vi "Write metadata to tiff string.vi"(8 "error in":errorcluster, 10 "Tiff image (unsigned byte array)":u8[](array[numeric]), 11 "Metadata string\n(must be at least 5 char long)":string) -> (0 "error out":errorcluster, 2 "Tiff file out (unsigned byte array)":u8[](array[numeric]))   [LabVIEW 2013, in "Tiff reader.lvlib"]
doc: "This .vi adds metadata to the tiff file (represented as a string)."
uses:
  Tiff reader.lvlib
  IFD Entry.ctl
  FieldTypes.ctl
  Long word to bytes.vi
panel:
  out "Time elapsed (ms)":u32
  out "Tag already exists?":bool
  out "Tag for metadata":T1
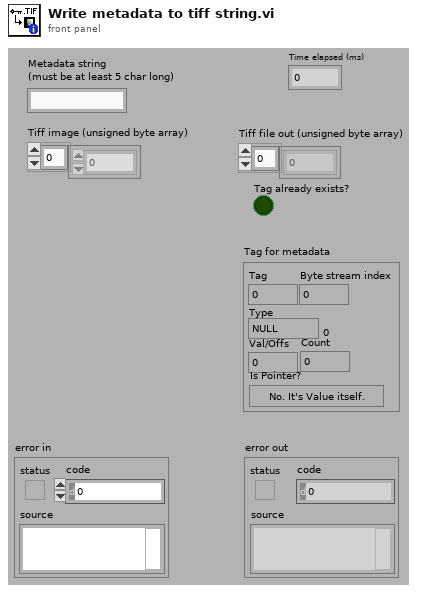
[diagram p1: front panel]
types:
  T1 = typedef "Tiff reader.lvlib/IFD Entry.ctl" = cluster{"Tag":u16, "Type":T2, "Count":u32, "Val/Offs":u32, "Is Pointer?":bool, "Byte stream index":i32}
  T2 = typedef "Tiff reader.lvlib/FieldTypes.ctl" = enum16{"NULL", "U8", "ASCII7", "U16", "U32", "RATIONAL", "SByte(I8)", "Undef(8Bit)", "I16", "I32", "SRat(4B:4B)", "SGL(4Byte)", "DBL(8Byte)"}
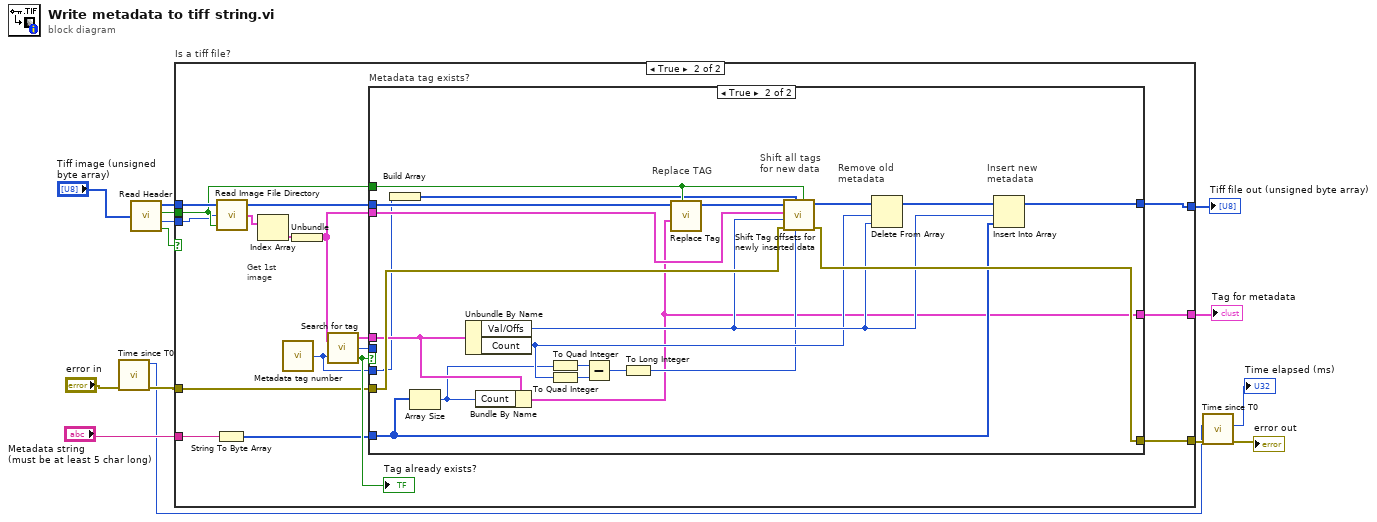
[diagram p0: block diagram]
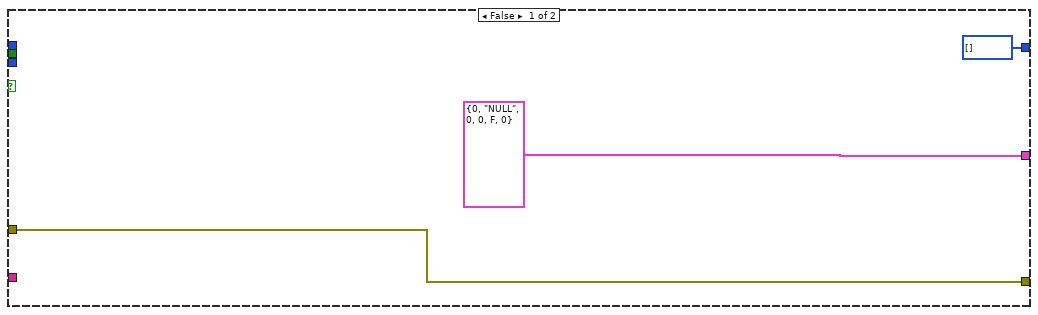
[diagram p2: hidden frame]
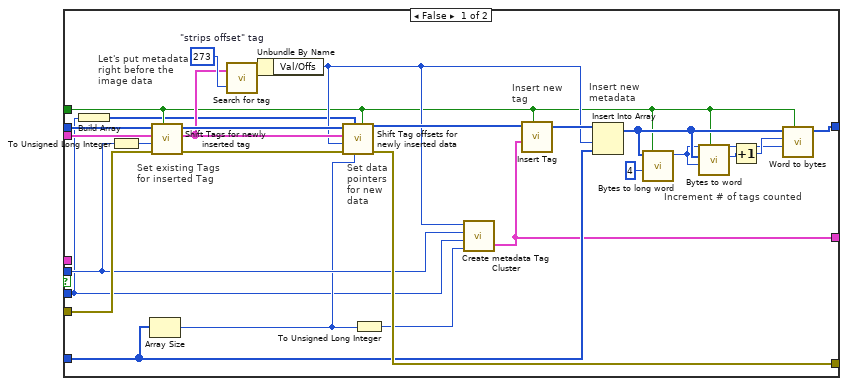
[diagram p3: hidden frame]
diagram:
  n1 = call "Time since T0.vi"("error in (no error)"="error in") -> ("error out"=w6:errorcluster, "current ms"=w2:u32)  [unwired: 2 in, 3 out]
  n2 = call "Read Header.vi"("TIFF Data in"="Tiff image (unsigned byte array)") -> ("TIFF Data out"=w13:u8[], "Litt/BigEnd"=w12:bool, "ImFileDirectOffs"=w14:u32, "IsTIFF?"=w11:bool)
  n3 = case "Is a tiff file?" shown="True" w11 {
    tunnel: w14 -> [_ w24]
    tunnel: w13 -> [_ w33]
    tunnel: [u8[] [] ("Image Data Out") w18] -> w9
    tunnel: w12 -> [_ w29]
    tunnel: "Metadata string\n(must be at least 5 char long)" -> [_ w27]
    tunnel: [T1 {"Tag"=0, "Type"=enum."NULL", "Count"=0, "Val/Offs"=0, "Is Pointer?"=FALSE, "Byte stream index"=0} ("Tag found") w25] -> w8
    tunnel: w6 -> [w16 w21]
    tunnel: [w16 w20] -> w5
    frame False {
    }
    frame True {
      # "Get 1st\nimage"
      n4 = String To Byte Array(string=w27) -> (unsigned byte array=w26:u8[])
      n5 = call "Read Image File Directory.vi"("Litt/BigEnd"=w29, "Im_File_Dir Offs"=w24, "Image Data in"=w33) -> ("Directories"=w34:cluster{"Tags":T1[]}[], "Image Data out"=w30:u8[])  [unwired: 1 out]
      n6 = Index Array(array=w34) -> (element=w23:cluster{"Tags":T1[]})  [unwired: 1 in]
      n7 = call "Metadata tag number.vi"() -> ("Tag to store\nmetadata in\n(ImageID tag)"=w19:u16)
      n8 = Unbundle(w23) -> ("Tags"=w22:T1[])
      n9 = call "Search for tag.vi"("Directory"=w22, "Tag"=w19) -> ("Tag found"=w32:T1, "Byte stream offset\nwhere tag should be"=w28:i32, "Tag exists?"=w31:bool)
      "Tag already exists?" <- w31
      n10 = case "Metadata tag exists?" shown="True" w31 {
        tunnel: w32 -> [_ w79]
        tunnel: w26 -> [w57 w78]
        tunnel: w30 -> [w53 w72]
        tunnel: w29 -> [w37 w71]
        tunnel: w22 -> [w56 w77]
        tunnel: w28 -> [w49 _]
        tunnel: [w41 w74] -> w18
        tunnel: w19 -> [w36 w63]
        tunnel: [w46 w64] -> w25
        tunnel: w21 -> [w61 w82]
        tunnel: [w60 w81] -> w20
        frame False {
          w55 = u16 273  # "strips offset" tag
          # "Increment # of tags counted"
          # "Set data \npointers\nfor new \ndata"
          # "Set existing Tags\nfor inserted Tag"
          # "Insert new \ntag"
          # "Insert new \nmetadata"
          # "Let's put metadata \nright before the \nimage data"
          n11 = Build Array(w36) -> (w35:u16[])
          n12 = To Unsigned Long Integer(number=w49) -> (unsigned 32bit integer=w48:u32)
          n13 = Array Size(array=w57) -> (size(s)=w45:i32)
          n14 = call "Shift Tags for newly inserted tag.vi"("Litt/BigEnd"=w37, "error in"=w61, "Byte stream offset\nwhere new tag added"=w48, "Directories"=w56, "Image Data"=w53) -> ("error out"=w59:errorcluster, "Directories out"=w50:T1[], "Image Data Out"=w58:u8[])  [unwired: 1 in, 1 out]
          n15 = call "Search for tag.vi"("Directory"=w50, "Tag"=w55) -> ("Tag found"=w54:T1)  [unwired: 2 out]
          n16 = Unbundle By Name(w54) -> ("Val/Offs"=w47:u32)
          n17 = call "Shift Tag offsets for newly inserted data.vi"("Litt/BigEnd"=w37, "Amount of data added\n(<0 means # of data bytesremoved)"=w45, "Ignore Tags"=w35, "error in"=w59, "Byte stream offset\nwhere new data added"=w47, "Directories"=w50, "Image Data"=w58) -> ("error out"=w60:errorcluster, "Image Data Out"=w52:u8[])  [unwired: 2 out]
          n18 = To Unsigned Long Integer(number=w45) -> (unsigned 32bit integer=w44:u32)
          n19 = call "Create metadata Tag Cluster.vi"("Count"=w44, "Tag to store\nmetadata in\n(ImageID tag)"=w36, "Byte stream offset\nwhere tag should have been"=w49, "Byte stream offset\nwhere data should be"=w47) -> ("Cluster"=w46:T1)  [unwired: 1 out]
          n20 = call "Insert Tag.vi"("Image Data in"=w52, "Cluster"=w46, "Litt/BigEnd"=w37) -> ("Image Data Out"=w51:u8[])  [unwired: 4 out]
          n21 = Insert Into Array(array=w51, index=w47, new element=w57) -> (w39:u8[])
          n22 = call "Bytes to long word.vi"("Litt/BigEnd"=w37, "Index"=4, "Image Data in"=w39) -> ("U32"=w38:u32)  [unwired: 6 out]
          n23 = call "Bytes to word.vi"("Litt/BigEnd"=w37, "Index"=w38, "Image Data in"=w39) -> ("Word"=w43:u16)  [unwired: 1 in, 5 out]
          n24 = Increment(x=w43) -> (x+1=w42:u16)
          n25 = call "Word to bytes.vi"("Litt/BigEnd"=w37, "Index"=w38, "Word"=w42, "Image Data in"=w39) -> ("Image Data out"=w41:u8[])  [unwired: 5 out]
        }
        frame True {
          # "Shift all tags\nfor new data"
          # "Replace TAG"
          # "Insert new \nmetadata"
          # "Remove old \nmetadata"
          n26 = Build Array(w63) -> (w62:u16[])
          n27 = Array Size(array=w78) -> (size(s)=w68:i32)
          n28 = Unbundle By Name(w79) -> ("Val/Offs"=w76:u32, "Count"=w69:u32)
          n29 = Bundle By Name(cluster=w79, "Count"=w68) -> (w64:T1)
          n30 = To Quad Integer(1:w68) -> (0:w67:i64)
          n31 = To Quad Integer(1:w69) -> (0:w70:i64)
          n32 = Subtract(x=w67, y=w70) -> (x-y=w66:i64)
          n33 = To Long Integer(number=w66) -> (32bit integer=w65:i32)
          n34 = call "Replace Tag.vi"("Litt/BigEnd"=w71, "Tag"=w64, "Image Data in"=w72) -> ("Image Data Out"=w73:u8[])  [unwired: 3 in, 2 out]
          n35 = call "Shift Tag offsets for newly inserted data.vi"("Litt/BigEnd"=w71, "Amount of data added\n(<0 means # of data bytesremoved)"=w65, "Ignore Tags"=w62, "error in"=w82, "Byte stream offset\nwhere new data added"=w76, "Directories"=w77, "Image Data"=w73) -> ("error out"=w81:errorcluster, "Image Data Out"=w75:u8[])  [unwired: 2 out]
          n36 = Delete From Array(array=w75, length=w69, index=w76) -> (array with subset deleted=w80:u8[])  [unwired: 1 out]
          n37 = Insert Into Array(array=w80, index=w76, new element=w78) -> (w74:u8[])
        }
      }
    }
  }
  "Tiff file out (unsigned byte array)" <- w9
  "Tag for metadata" <- w8
  n38 = call "Time since T0.vi"("error in (no error)"=w5, "T0 millisecond timer value"=w2) -> ("error out"=→"error out":errorcluster, "Time elapsed (ms)"=→"Time elapsed (ms)":u32)  [unwired: 1 in, 3 out]
